vi "StageMiniUI.vi"() -> ()   [LabVIEW 2017]
uses:
  AEROTECstageAPI/SingleStageData.ctl
  AEROTECstageAPI/StageEnum.ctl
  AEROTECstageAPI/MoveDistanceInAxis.ctl
  Utility/Axis Direction Definition.ctl
panel:
  in  "Disable Stage":bool
  in  "Distance (microns)":dbl
  in  "Left Button":bool
  in  "Right Button":bool
  in  "Down Button":bool
  in  "Up Button":bool
  in  "Enable Stage":bool
  out "Stage Data":T1[](array[typedef])
  out "error out":errorcluster
  in  "stop 2":bool
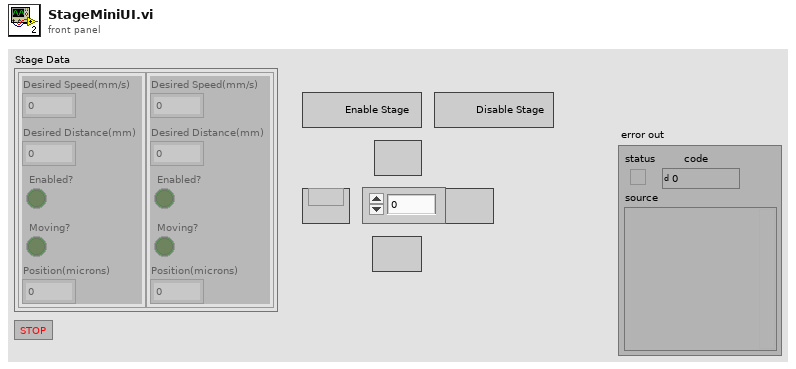
[diagram p1: front panel]
types:
  T1 = typedef "SingleStageData.ctl" = cluster{"Desired Speed(mm/s)":dbl, "Desired Distance(mm)":dbl, "Enabled?":bool, "Moving?":bool, "Position(microns)":dbl}
  T2 = typedef "StageEnum.ctl" = enum16{"Get Current Pos!", "Move axis!", "Enable Stage!", "Stop Stage Controller!", "Set Default Speeds!", "Get Stage Parameters", "Start Stage Controller!", "Init", "Go Home!"}
  T3 = typedef "Axis Direction Definition.ctl" = enum16{"Axis left/right", "Axis up/down"}
  T4 = typedef "MoveDistanceInAxis.ctl" = cluster{"Axis Number":i16, "Distance (microns)":dbl}
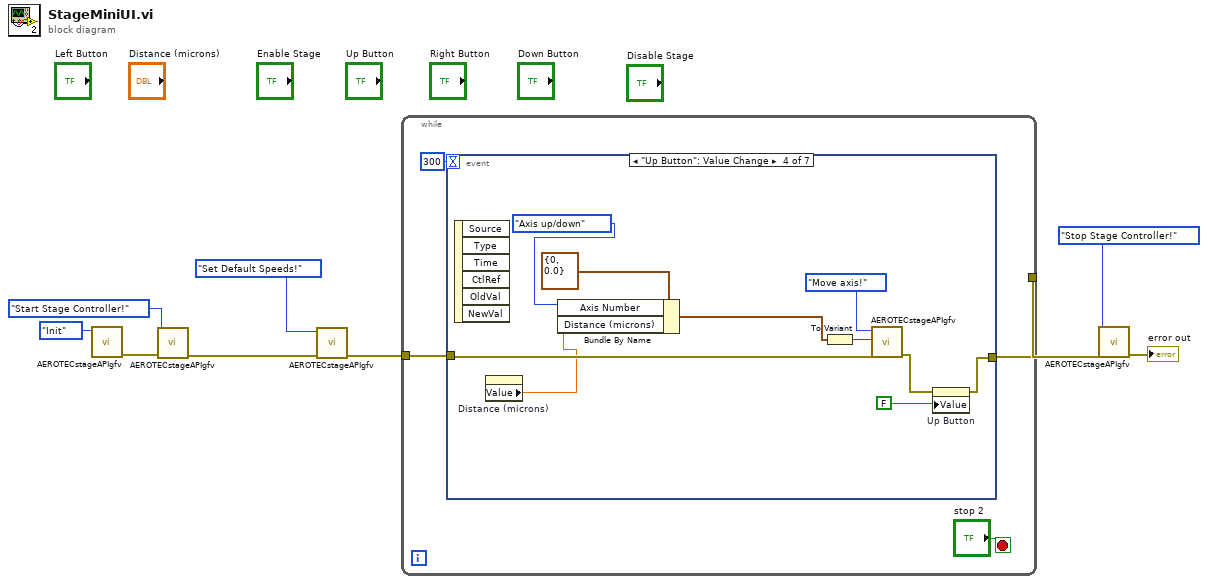
[diagram p0: block diagram]
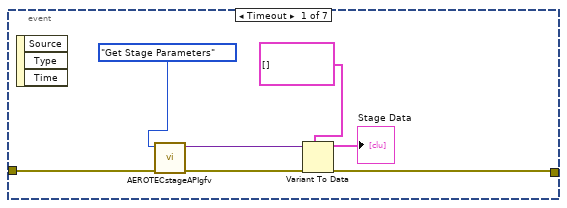
[diagram p2: hidden frame]
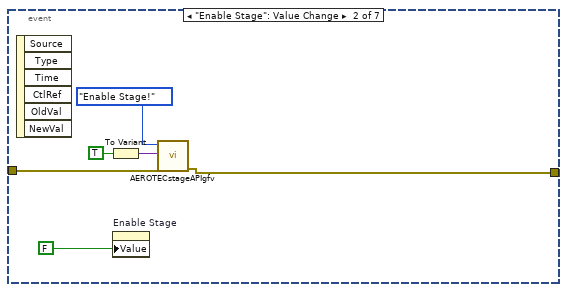
[diagram p3: hidden frame]
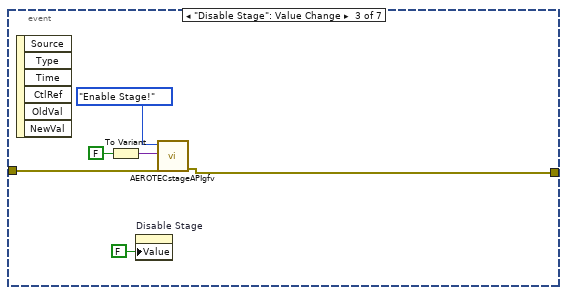
[diagram p4: hidden frame]
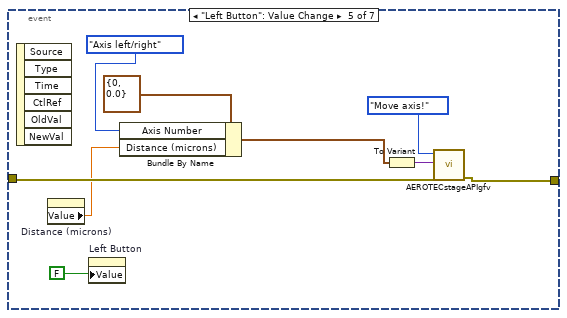
[diagram p5: hidden frame]
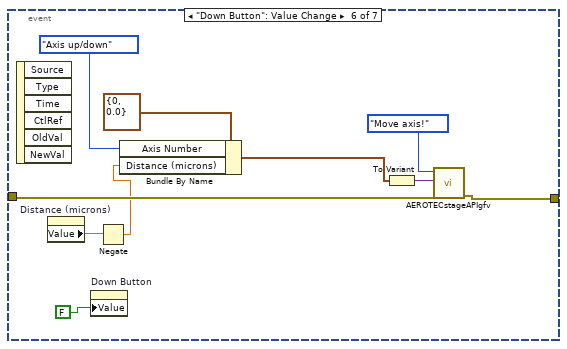
[diagram p6: hidden frame]
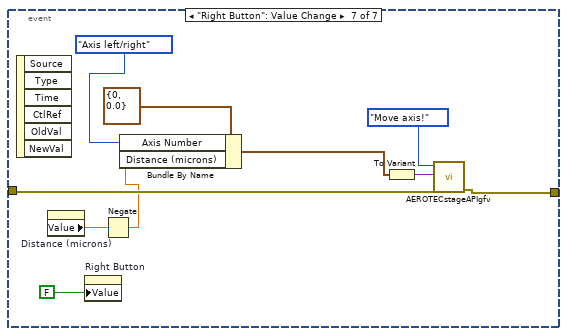
[diagram p7: hidden frame]
diagram:
  n1 = call "AEROTECstageAPIgfv.vi"("StageContrlEnum"=StageEnum."Init") -> ("error out"=w8:errorcluster)  [unwired: 9 in, 1 out]
  n2 = call "AEROTECstageAPIgfv.vi"("error in (no error)"=w8, "StageContrlEnum"=StageEnum."Start Stage Controller!") -> ("error out"=w4:errorcluster)  [unwired: 8 in, 1 out]
  n3 = call "AEROTECstageAPIgfv.vi"("error in (no error)"=w4, "StageContrlEnum"=StageEnum."Set Default Speeds!") -> ("error out"=w2:errorcluster)  [unwired: 8 in, 1 out]
  n4 = while {
    tunnel: w2 -> [w11]
    tunnel: [w10] -> w1
    stop <- "stop 2" stop-if-true
    n5 = event shown="[3] \"Up Button\": Value Change" {
      selector: _ -> [_ _ _ _ _ _ _]
      dyn-events: _ -> [_ _ _ _ _ _ _]
      timeout: 300 -> [_ _ _ _ _ _ _]
      tunnel: w11 -> [w16 w25 w31 w41 w50 w60 w70]
      tunnel: [w14 w24 w30 w34 w49 w59 w69] -> w10
      event Timeout {
        n6 = event-data() -> ()  [unwired: 1 in, 3 out]
        n7 = call "AEROTECstageAPIgfv.vi"("error in (no error)"=w16, "StageContrlEnum"=StageEnum."Get Stage Parameters") -> ("error out"=w14:errorcluster, "Data Out"=w19:variant)  [unwired: 8 in]
        n8 = Variant To Data(type=T1[] [], Variant=w19) -> (data=→"Stage Data":T1[])  [unwired: 1 in, 1 out]
      }
      event "Enable Stage": Value Change {
        n9 = event-data() -> ()  [unwired: 1 in, 6 out]
        n10 = To Variant(anything=TRUE) -> (Variant=w21:variant)
        n11 = property on="Enable Stage" class="Bool (strict)"("Value"=FALSE) -> ()  [unwired: 2 in, 2 out]
        n12 = call "AEROTECstageAPIgfv.vi"("error in (no error)"=w25, "Data in"=w21, "StageContrlEnum"=StageEnum."Enable Stage!") -> ("error out"=w24:errorcluster)  [unwired: 7 in, 1 out]
      }
      event "Disable Stage": Value Change {
        n13 = event-data() -> ()  [unwired: 1 in, 6 out]
        n14 = To Variant(anything=FALSE) -> (Variant=w27:variant)
        n15 = property on="Disable Stage" class="Bool (strict)"("Value"=FALSE ("Disable Stage")) -> ()  [unwired: 2 in, 2 out]
        n16 = call "AEROTECstageAPIgfv.vi"("error in (no error)"=w31, "Data in"=w27, "StageContrlEnum"=StageEnum."Enable Stage!") -> ("error out"=w30:errorcluster)  [unwired: 7 in, 1 out]
      }
      event "Up Button": Value Change {
        n17 = event-data() -> ()  [unwired: 1 in, 6 out]
        n18 = property on="Distance (microns)" class="DigNum (strict)"() -> ("Value"=w32:dbl)  [unwired: 2 in, 2 out]
        n19 = Bundle By Name(cluster=T4 {"Axis Number"=0, "Distance (microns)"=0.0} ("MoveDistanceInAxis"), "Axis Number"=Axis_Direction_Definition."Axis up/down", "Distance (microns)"=w32) -> (w37:T4)
        n20 = To Variant(anything=w37) -> (Variant=w39:variant)
        n21 = call "AEROTECstageAPIgfv.vi"("error in (no error)"=w41, "Data in"=w39, "StageContrlEnum"=StageEnum."Move axis!") -> ("error out"=w35:errorcluster)  [unwired: 7 in, 1 out]
        n22 = property on="Up Button" class="Bool (strict)"(error in=w35, "Value"=FALSE ("Disable Stage")) -> (error out=w34:errorcluster)  [unwired: 1 in, 1 out]
      }
      event "Left Button": Value Change {
        n23 = event-data() -> ()  [unwired: 1 in, 6 out]
        n24 = property on="Distance (microns)" class="DigNum (strict)"() -> ("Value"=w42:dbl)  [unwired: 2 in, 2 out]
        n25 = property on="Left Button" class="Bool (strict)"("Value"=FALSE ("Disable Stage")) -> ()  [unwired: 2 in, 2 out]
        n26 = Bundle By Name(cluster=T4 {"Axis Number"=0, "Distance (microns)"=0.0} ("MoveDistanceInAxis"), "Axis Number"=Axis_Direction_Definition."Axis left/right", "Distance (microns)"=w42) -> (w45:T4)
        n27 = To Variant(anything=w45) -> (Variant=w47:variant)
        n28 = call "AEROTECstageAPIgfv.vi"("error in (no error)"=w50, "Data in"=w47, "StageContrlEnum"=StageEnum."Move axis!") -> ("error out"=w49:errorcluster)  [unwired: 7 in, 1 out]
      }
      event "Down Button": Value Change {
        n29 = event-data() -> ()  [unwired: 1 in, 6 out]
        n30 = property on="Distance (microns)" class="DigNum (strict)"() -> ("Value"=w52:dbl)  [unwired: 2 in, 2 out]
        n31 = property on="Down Button" class="Bool (strict)"("Value"=FALSE ("Disable Stage")) -> ()  [unwired: 2 in, 2 out]
        n32 = Negate(x=w52) -> (-x=w51:dbl)
        n33 = Bundle By Name(cluster=T4 {"Axis Number"=0, "Distance (microns)"=0.0} ("MoveDistanceInAxis"), "Axis Number"=Axis_Direction_Definition."Axis up/down", "Distance (microns)"=w51) -> (w55:T4)
        n34 = To Variant(anything=w55) -> (Variant=w57:variant)
        n35 = call "AEROTECstageAPIgfv.vi"("error in (no error)"=w60, "Data in"=w57, "StageContrlEnum"=StageEnum."Move axis!") -> ("error out"=w59:errorcluster)  [unwired: 7 in, 1 out]
      }
      event "Right Button": Value Change {
        n36 = event-data() -> ()  [unwired: 1 in, 6 out]
        n37 = property on="Distance (microns)" class="DigNum (strict)"() -> ("Value"=w62:dbl)  [unwired: 2 in, 2 out]
        n38 = property on="Right Button" class="Bool (strict)"("Value"=FALSE ("Disable Stage")) -> ()  [unwired: 2 in, 2 out]
        n39 = Negate(x=w62) -> (-x=w61:dbl)
        n40 = Bundle By Name(cluster=T4 {"Axis Number"=0, "Distance (microns)"=0.0} ("MoveDistanceInAxis"), "Axis Number"=Axis_Direction_Definition."Axis left/right", "Distance (microns)"=w61) -> (w65:T4)
        n41 = To Variant(anything=w65) -> (Variant=w67:variant)
        n42 = call "AEROTECstageAPIgfv.vi"("error in (no error)"=w70, "Data in"=w67, "StageContrlEnum"=StageEnum."Move axis!") -> ("error out"=w69:errorcluster)  [unwired: 7 in, 1 out]
      }
    }
  }
  n43 = call "AEROTECstageAPIgfv.vi"("error in (no error)"=w1, "StageContrlEnum"=StageEnum."Stop Stage Controller!") -> ("error out"=→"error out":errorcluster)  [unwired: 8 in, 1 out]
